vi "Reserve Sessions - 1 Pin.vi"(6 "timeout (ms)":i32, 8 "error in (no error)":errorcluster, 10 "pin or relay name":string, 11 "measurement context in":refnum<class "MeasurementContext.lvclass">) -> (0 "error out":errorcluster, 2 "session reservation out":refnum<class "Session Reservation.lvclass">, 3 "measurement context out":refnum<class "MeasurementContext.lvclass">)   [LabVIEW 2020, in "MeasurementLink Measurement Server.lvlib" / "MeasurementContext.lvclass"]
doc: "Reserves session(s) based on the provided pin information."
uses:
  MeasurementContext.lvclass
  MeasurementLink Session Management/Session Reservation/Session Reservation.lvclass
  MeasurementContext.lvclass/MeasurementContext.ctl
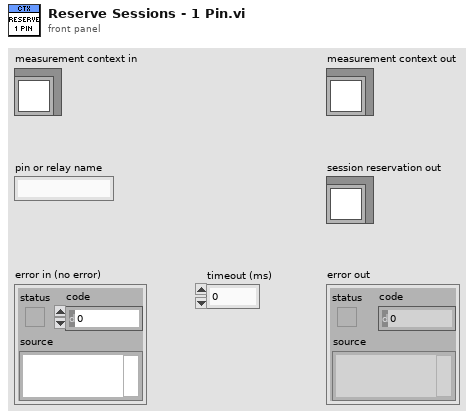
[diagram p1: front panel]
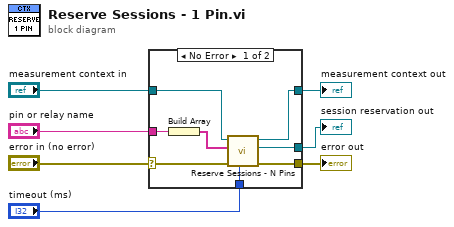
[diagram p0: block diagram]
diagram:
  n1 = case shown="No Error" "error in (no error)" {
    selector: "error in (no error)" -> [w13 w17]
    tunnel: [w9 w17] -> w6
    tunnel: [w14 w16] -> w4
    tunnel: "measurement context in" -> [w15 w16]
    tunnel: "pin or relay name" -> [w11 _]
    tunnel: "timeout (ms)" -> [w8 _]
    tunnel: [w10 _] -> w1
    frame No Error {
      n2 = Build Array(w11) -> (w12:string[])
      n3 = call "Reserve Sessions - N Pins.vi"("timeout (ms)"=w8, "error in (no error)"=w13, "pin or relay names"=w12, "measurement context in"=w15) -> ("error out"=w9:errorcluster, "session reservation out"=w10:refnum<class "Session Reservation.lvclass">, "measurement context out"=w14:refnum<class "MeasurementContext.lvclass">)  [unwired: 5 in]
    }
    frame Error {
    }
  }
  "error out" <- w6
  "measurement context out" <- w4
  "session reservation out" <- w1
